vi "String To Enum.vi"(8 "error in (no error)":errorcluster, 11 "string":string) -> (0 "error out":errorcluster, 3 "Select Update Rate":enum16{"HIGH", "MEDIUM", "LOW"}(ring))   [LabVIEW 2019, in "Zen Analytics.lvlib" / "Zen Analytics.lvclass"]
uses:
  Zen Analytics.lvclass
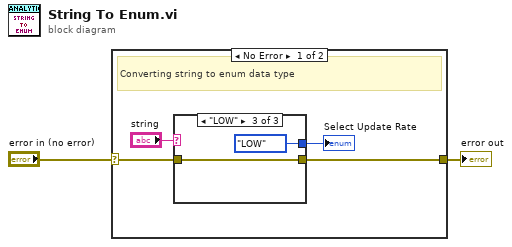
[diagram p0: block diagram]
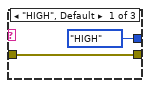
[diagram p2: hidden frame]
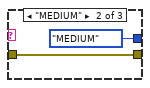
[diagram p3: hidden frame]
diagram:
  n1 = case shown="No Error" "error in (no error)" {
    selector: "error in (no error)" -> [w6 w13]
    tunnel: [w5 w13] -> w1
    frame No Error {
      # "Converting string to enum data type"
      n2 = case shown="\"LOW\"" "string" {
        tunnel: w6 -> [w7 w9 w12]
        tunnel: [w7 w9 w12] -> w5
        tunnel: [enum16{"HIGH", "MEDIUM", "LOW"}."HIGH" ("Select Update Rate") enum16{"HIGH", "MEDIUM", "LOW"}."MEDIUM" ("Select Update Rate") enum16{"HIGH", "MEDIUM", "LOW"}."LOW" ("Select Update Rate")] -> w3
        frame "HIGH", Default {
        }
        frame "MEDIUM" {
        }
        frame "LOW" {
        }
      }
      "Select Update Rate" <- w3
    }
    frame Error {
    }
  }
  "error out" <- w1
